vi "Initialize Attributes.vi"(8 "error in (no error)":errorcluster, 10 "Attribute Data":variant, 11 "Example in":refnum<class "Example.lvclass">) -> (0 "error out":errorcluster, 2 "Found?":bool, 3 "Example out":refnum<class "Example.lvclass">)   [LabVIEW 2013, in "CS++Core-Examples.lvlib" / "Example.lvclass"]
doc: "Initialize object attribute.\n\nUnique resources should be allocated elsewhere!"
uses:
  Example.lvclass
  Core/Classes/CS++BaseClasses/Base/CS++Base.lvclass
  Example.lvclass/Example.ctl
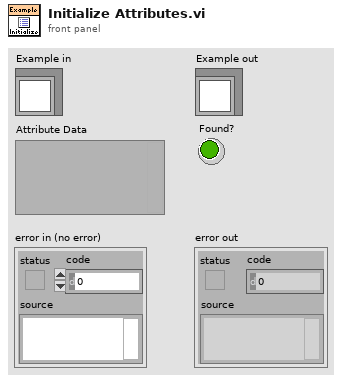
[diagram p1: front panel]
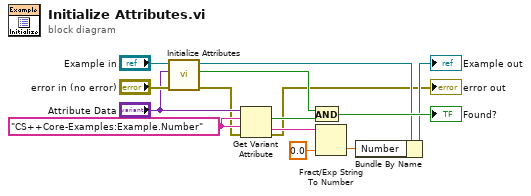
[diagram p0: block diagram]
diagram:
  w7 = "CS++Core-Examples:Example.Number" ("name")
  n1 = call-parent "Initialize Attributes.vi"("error in (no error)"="error in (no error)", "Attribute Data"="Attribute Data", "CS++Base in"="Example in") -> ("error out"=w2:errorcluster, "Found?"=w14:bool, "CS++Base out"=w4:refnum<class "Example.lvclass">)  [unwired: 6 in]
  n2 = Get Variant Attribute(Variant="Attribute Data", name=w7, default value (empty Variant)=w7, error in=w2) -> (found=w9:bool, value=w8:string, error out=→"error out":errorcluster)  [unwired: 1 out]
  n3 = And(x=w14, y=w9) -> (x .and. y?=→"Found?":bool)
  n4 = Fract/Exp String To Number(string=w8, default (0 dbl)=0.0 ("default (0 DBL)")) -> (number=w5:dbl)  [unwired: 2 in, 1 out]
  n5 = Bundle By Name(cluster=w4, "Number"=w5) -> (→"Example out":refnum<class "Example.lvclass">)
